vi "Assert Warning.vi"(4 "Execution time (s)":dbl=-1.0, 6 "error code (1)":i32=1, 7 "Label":string, 8 "error in":errorcluster, 11 "warning":errorcluster) -> (0 "error out":errorcluster, 2 "Properties":refnum<class "Properties.Assert.lvclass">)   [LabVIEW 2021, in "Banana.Caraya.lvlib" / "Platano.CarayaTestSuite.lvclass"]
uses:
  Banana.Caraya/Platano.CarayaTestSuite/Platano.CarayaTestSuite.lvclass
  Banana.Caraya/Platano.CarayaTestSuite/Platano.CarayaTestSuite.lvclass/Platano.CarayaTestSuite.ctl
  <vilib>/addons/_JKI Toolkits/Caraya/classes/Assert/Assert.lvclass
  Platano/Platano.lvclass
  Banana/Banana.lvclass
  <vilib>/addons/_JKI Toolkits/Caraya/classes/Assert/Assert True.vi
  AssetError/AssertError.lvclass
  Banana.Caraya/Properties.Banana/Properties.Banana.lvclass
  <vilib>/addons/_JKI Toolkits/Caraya/classes/Properties.Assert/Properties.Assert.lvclass
  C:/Program Files (x86)/National Instruments/LabVIEW 2021/vi.lib/addons/_JKI Toolkits/Caraya/classes/Properties/Properties.lvclass
  C:/Program Files (x86)/National Instruments/LabVIEW 2021/vi.lib/addons/_JKI Toolkits/Caraya/classes/Properties.Assert/Properties.Assert.lvclass
  C:/Repositories/LVOS/Bananas/lv-src/Bananas/AssetError/AssertError.lvclass
  C:/Repositories/LVOS/Bananas/lv-src/Bananas/BananaPeel/BananaPeel.lvclass
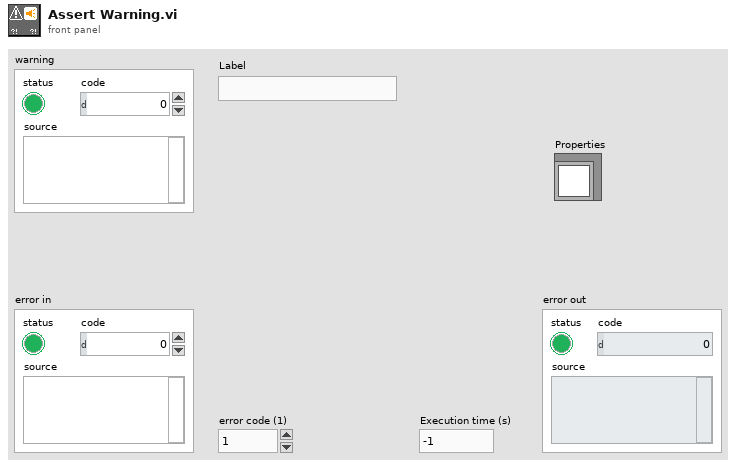
[diagram p1: front panel]
types:
  T1 = typedef "Bananas.lvlib/Assertion Strategies -- cluster.ctl" = cluster{"AssertTrue":refnum<class "AssertTrue.lvclass">, "AssertFalse":refnum<class "AssertFalse.lvclass">, "AssertEqualValue":refnum<class "AssertEqualValue.lvclass">, "AssertEqualType":refnum<class "AssertEqualType.lvclass">, "AssertCompareValue":refnum<class "AssertCompareValue.lvclass">, "AssertError":refnum<class "AssertError.lvclass">, "AssertAlmostEqual":refnum<class "AssertAlmostEqualValue.lvclass">}
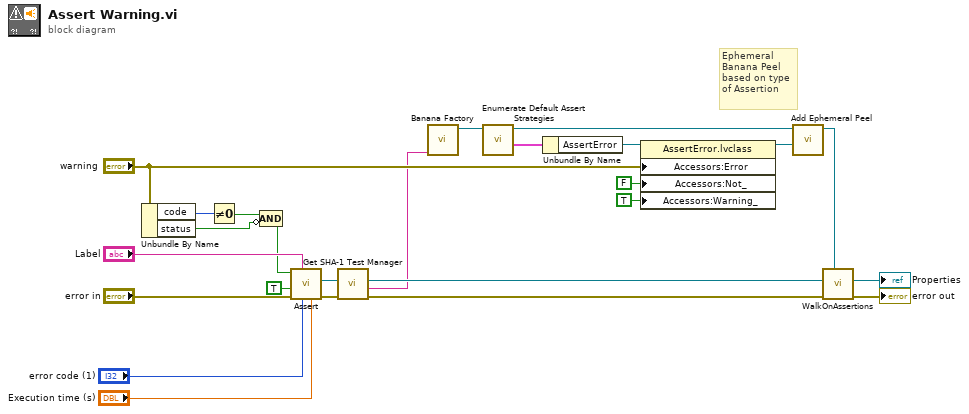
[diagram p0: block diagram]
diagram:
  # "Ephemeral\nBanana Peel\nbased on type\nof Assertion"
  n1 = Unbundle By Name("warning") -> ("code"=w10:i32, "status"=w8:bool)
  n2 = Not Equal To 0?(x=w10) -> (x != 0?=w9:bool)
  n3 = Compound Arithmetic op=AND(w9, invert w8) -> (w7:bool)
  n4 = call-poly <vilib>:"Assert.vi"("Execution time (s)"="Execution time (s)", "error code (1)"="error code (1)", "Label"="Label", "error in (no error)"="error in", "Register with caller test (F)"=TRUE, "True?"=w7) -> ("error out"=w6:errorcluster, "Properties"=w4:refnum<class "Properties.Assert.lvclass">)  [unwired: 4 in]
  n5 = call "Get SHA-1 Test Manager.vi"("error in (no error)"=w6, "Properties"=w4) -> ("error out"=w5:errorcluster, "SHA-1 hash"=w2:string, "Properties"=w3:refnum<class "Properties.Assert.lvclass">)  [unwired: 7 in]
  n6 = call "Banana Factory.vi"("Varietal"=w2) -> ("Banana"=w1:refnum<class "Banana.lvclass">)  [unwired: 10 in]
  n7 = call "Enumerate Default Assert Strategies.vi"("Banana"=w1) -> ("Strategies"=w16:T1, "Banana"=w17:refnum<class "Banana.lvclass">)  [unwired: 9 in]
  n8 = Unbundle By Name(w16) -> ("AssertError"=w15:refnum<class "AssertError.lvclass">)
  n9 = property class="AssertError.lvclass"(reference=w15, "Accessors:Error"="warning", "Accessors:Not_"=FALSE ("Not_"), "Accessors:Warning_"=TRUE ("Warning_")) -> (reference out=w14:refnum<class "AssertError.lvclass">)  [unwired: 1 in, 1 out]
  n10 = call "Add Ephemeral Peel.vi"("BananaPeel"=w14, "Banana"=w17) -> ("Banana"=w18:refnum<class "Banana.lvclass">)  [unwired: 8 in, 1 out]
  n11 = call "WalkOnAssertions.vi"("Banana"=w18, "error in (no error)"=w5, "Properties"=w3) -> ("error out"=→"error out":errorcluster, "Properties out"=→"Properties":refnum<class "Properties.Assert.lvclass">)  [unwired: 7 in]
